vi "Configure Scaling.vi"(0 "VISA resource name":refnum<visa-resource-name>, 1 "Enable Scaling (T: Enable)":bool=TRUE, 2 "Element (0: All)":i32(ring) items=["All", "1", "2", "3"], 5 "VT Ratio (1.000)":dbl=1.0 min=0.001 max=9999.999 format="%.3g", 7 "CT Ratio (1.000)":dbl=1.0 min=0.001 max=9999.999 format="%.3g", 9 "Power Coefficient (1.000)":dbl=1.0 min=0.001 max=9999.999 format="%.3g", 11 "error in (no error)":errorcluster) -> (4 "VISA resource name out":refnum<visa-resource-name>, 15 "error out":errorcluster)   [LabVIEW 2016, in "Yokogawa WT300 Series.lvlib"]
doc: "Configures the scaling features."
uses:
  Yokogawa WT300 Series.lvlib
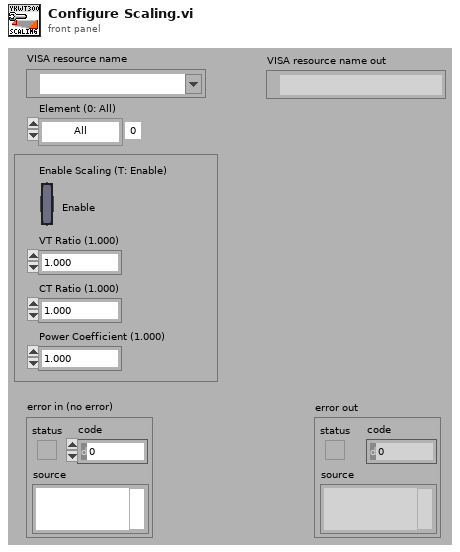
[diagram p1: front panel]
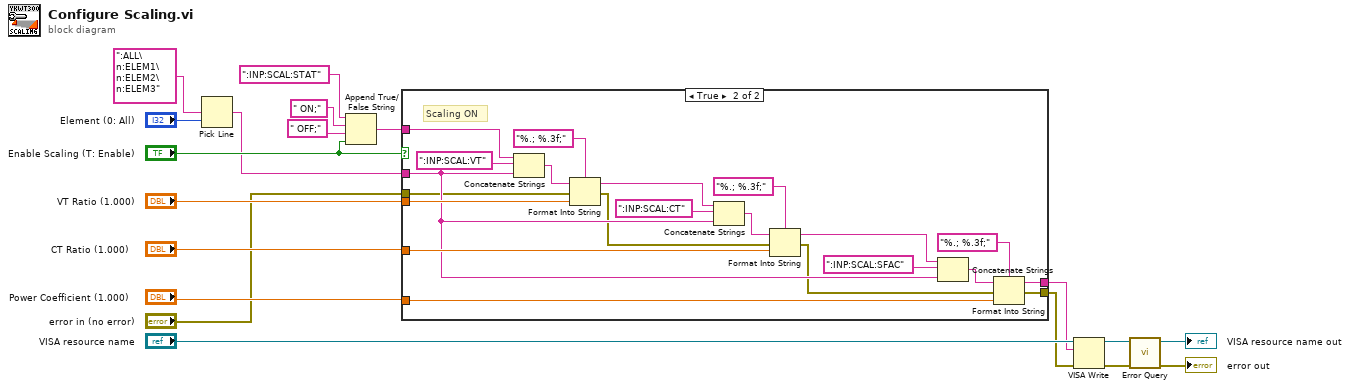
[diagram p0: block diagram]
diagram:
  n1 = Pick Line ("ライン選択")(multi-line string=":ALL\n:ELEM1\n:ELEM2\n:ELEM3" ("¡s¶ñ"), line index="Element (0: All)") -> (output string=w8:string)  [unwired: 1 in]
  n2 = Append True/False String ("True/False 文字列を追加")(1:"Enable Scaling (T: Enable)", 2:" OFF;", 3:" ON;", 4:":INP:SCAL:STAT") -> (0:w9:string)
  n3 = case "ケースストラクチャ" shown="True" "Enable Scaling (T: Enable)" {
    tunnel: w9 -> [w21 w40]
    tunnel: w8 -> [_ w28]
    tunnel: "VT Ratio (1.000)" -> [_ w38]
    tunnel: "CT Ratio (1.000)" -> [_ w33]
    tunnel: "Power Coefficient (1.000)" -> [_ w27]
    tunnel: "error in (no error)" -> [w20 w24]
    tunnel: [w21 w23] -> w3
    tunnel: [w20 w22] -> w2
    frame False {
      # "Scaling OFF"
    }
    frame True {
      # "Scaling ON"
      n4 = Concatenate Strings(w40, ":INP:SCAL:VT", w28) -> (w39:string)
      n5 = Format Into String ("文字列にフォーマット")(format string="%.; %.3f;" ("Œ`Ž®•¶Žš—ñ"), initial string=w39, error in=w24, w38) -> (resulting string=w34:string, error out=w25:errorcluster)
      n6 = Concatenate Strings(w34, ":INP:SCAL:CT", w28) -> (w37:string)
      n7 = Format Into String ("文字列にフォーマット")(format string="%.; %.3f;" ("Œ`Ž®•¶Žš—ñ"), initial string=w37, error in=w25, w33) -> (resulting string=w29:string, error out=w26:errorcluster)
      n8 = Concatenate Strings(w29, ":INP:SCAL:SFAC", w28) -> (w30:string)
      n9 = Format Into String ("文字列にフォーマット")(format string="%.; %.3f;" ("Œ`Ž®•¶Žš—ñ"), initial string=w30, error in=w26, w27) -> (resulting string=w23:string, error out=w22:errorcluster)
    }
  }
  n10 = VISA Write ("VISA書き込み")(VISA resource name="VISA resource name", write buffer=w3, error in (no error)=w2) -> (VISA resource name out=w19:refnum<visa-resource-name>, error out=w18:errorcluster)  [unwired: 1 out]
  n11 = call "Error Query.vi"("error in (no error)"=w18, "VISA resource name"=w19) -> ("error out"=→"error out":errorcluster, "VISA resource name out"=→"VISA resource name out":refnum<visa-resource-name>)  [unwired: 6 in, 2 out]
